vi "SDSU_DACS_parse_request.vi"(10 "desired points":string) -> (0 "number of points":i32, 1 "mult. points?":bool, 2 "names":string[](array[string]))   [LabVIEW 2016]
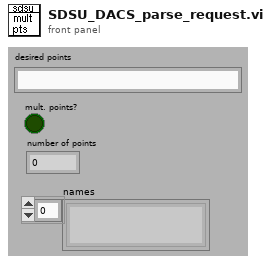
[diagram p1: front panel]
types:
  T1 = enum16{"read from file", "find", "set", "set_to_default", "get all"}
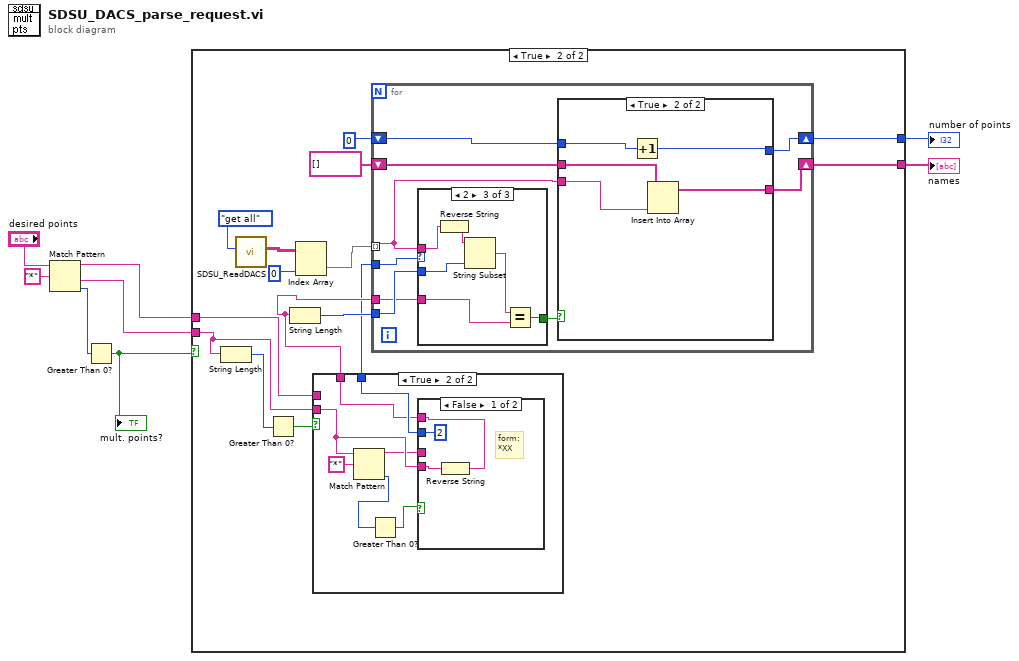
[diagram p0: block diagram]
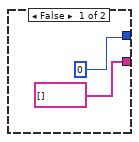
[diagram p2: hidden frame]
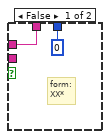
[diagram p3: hidden frame]
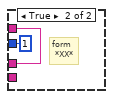
[diagram p4: hidden frame]
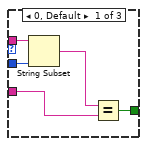
[diagram p5: hidden frame]
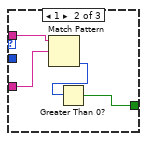
[diagram p6: hidden frame]
diagram:
  n1 = Match Pattern(string="desired points", regular expression="*") -> (before substring=w4:string, after substring=w1:string, offset past match=w6:i32)  [unwired: 2 out]
  n2 = Greater Than 0?(x=w6) -> (x > 0?=w5:bool)
  "mult. points?" <- w5
  n3 = case shown="True" w5 {
    tunnel: w4 -> [_ w13]
    tunnel: [0 w18] -> w3
    tunnel: [string[] [] w17] -> w2
    tunnel: w1 -> [_ w14]
    frame False {
    }
    frame True {
      n4 = String Length(string=w14) -> (length=w16:i32)
      n5 = call "SDSU_ReadDACS.vi"("action"=T1."get all") -> ("Table"=w24:string[][])  [unwired: 4 in, 6 out]
      n6 = Greater Than 0?(x=w16) -> (x > 0?=w15:bool)
      n7 = Index Array(array=w24, index (col)=0 ("index")) -> (element=w22:string[])  [unwired: 1 in]
      n8 = case shown="True" w15 {
        tunnel: w14 -> [_ w30]
        tunnel: w13 -> [w27 _]
        tunnel: [w27 w28] -> w12
        tunnel: [0 w31] -> w11
        frame False {
          # "form:\nXX*"
        }
        frame True {
          n9 = Match Pattern(string=w30, regular expression="*") -> (before substring=w29:string, offset past match=w33:i32)  [unwired: 3 out]
          n10 = Greater Than 0?(x=w33) -> (x > 0?=w32:bool)
          n11 = case shown="False" w32 {
            tunnel: [2 1] -> w31
            tunnel: w30 -> [w36 _]
            tunnel: w29 -> [_ w38]
            tunnel: [w35 w38] -> w28
            frame False {
              # "form:\n*XX"
              n12 = Reverse String(1:w36) -> (0:w35:string)
            }
            frame True {
              # "form\n *XX*"
            }
          }
        }
      }
      n13 = String Length(string=w12) -> (length=w21:i32)
      n14 = for {
        tunnel: w12 -> [w47]
        tunnel: w22 -> [w45] mode=indexing
        tunnel: w21 -> [w48]
        shift-right: [w43] -> w18
        shift-left: 0 -> [w44]
        shift-right: [w42] -> w17
        shift-left: string[] [] -> [w41]
        tunnel: w11 -> [w40]
        n15 = case shown="2" w40 {
          tunnel: w48 -> [w53 _ w61]
          tunnel: w47 -> [w52 w56 w59]
          tunnel: [w51 w54 w58] -> w46
          tunnel: w45 -> [w49 w57 w63]
          frame 0, Default {
            n16 = String Subset(string=w49, length (rest)=w53) -> (substring=w50:string)  [unwired: 1 out]
            n17 = Equal?(x=w50, y=w52) -> (x = y?=w51:bool)
          }
          frame 1 {
            n18 = Match Pattern(string=w57, regular expression=w56) -> (offset past match=w55:i32)  [unwired: 4 out]
            n19 = Greater Than 0?(x=w55) -> (x > 0?=w54:bool)
          }
          frame 2 {
            n20 = Reverse String(1:w63) -> (0:w62:string)
            n21 = String Subset(string=w62, length (rest)=w61) -> (substring=w60:string)  [unwired: 1 out]
            n22 = Equal?(x=w60, y=w59) -> (x = y?=w58:bool)
          }
        }
        n23 = case shown="True" w46 {
          tunnel: w45 -> [_ w68]
          tunnel: w44 -> [w65 w70]
          tunnel: [w65 w69] -> w43
          tunnel: [w64 w67] -> w42
          tunnel: w41 -> [w64 w66]
          frame False {
          }
          frame True {
            n24 = Increment(x=w70) -> (x+1=w69:i32)
            n25 = Insert Into Array(array=w66, new element=w68) -> (w67:string[])  [unwired: 1 in]
          }
        }
      }
    }
  }
  "number of points" <- w3
  "names" <- w2
